vi "get active handles.vi"(8 "error in (no error)":errorcluster, 11 "Hamamatsu Camera in":refnum<class "Hamamatsu Camera.lvclass">) -> (0 "error out":errorcluster, 1 "Active Cameras":T1[](array[typedef]), 2 "Handles":u32[](array[numeric]), 3 "Hamamatsu Camera out":refnum<class "Hamamatsu Camera.lvclass">, 5 "Camera Names":string[](array[string]))   [LabVIEW 2018, in "Hamamatsu Camera.lvlib" / "Hamamatsu Camera.lvclass"]
uses:
  Hamamatsu Camera.lvclass
  Resources/Type Defs/Physical Camera Assignment.ctl
  Resources/Type Defs/Camera Type.ctl
  Hamamatsu Camera.lvclass/Hamamatsu Camera.ctl
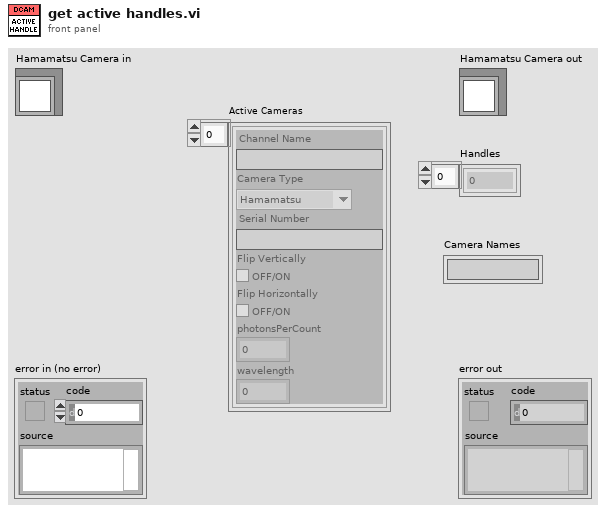
[diagram p1: front panel]
types:
  T1 = typedef "Physical Camera Assignment.ctl" = cluster{"Channel Name":string, "Camera Type":T2, "Serial Number":string, "Flip Vertically":bool, "Flip Horizontally":bool, "photonsPerCount":dbl, "wavelength":i16}
  T2 = typedef "Camera Type.ctl" = enum16{"Hamamatsu"}
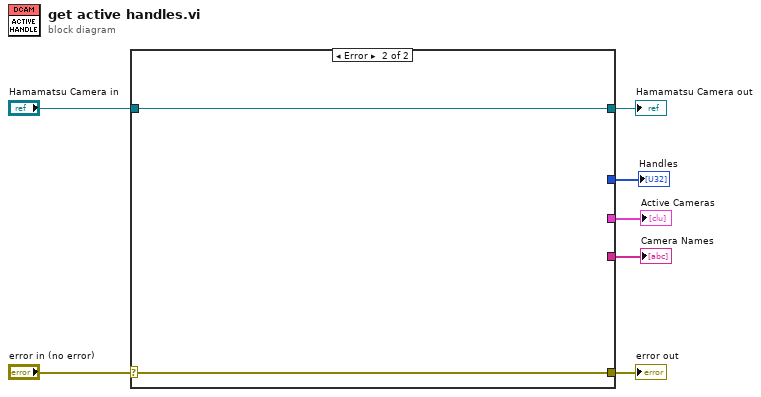
[diagram p0: block diagram]
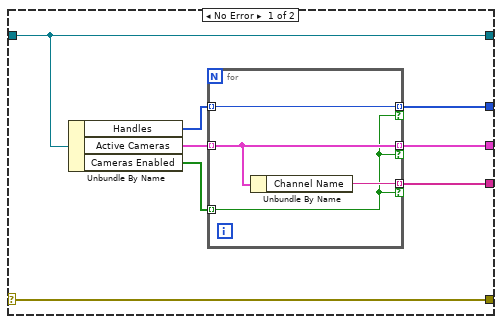
[diagram p2: hidden frame]
diagram:
  n1 = case shown="Error" "error in (no error)" {
    selector: "error in (no error)" -> [w15 w21]
    tunnel: [w15 w21] -> w6
    tunnel: [w14 w20] -> w4
    tunnel: "Hamamatsu Camera in" -> [w14 w20]
    tunnel: [w10 _] -> w3
    tunnel: [w9 _] -> w2
    tunnel: [w8 _] -> w1
    frame No Error {
      n2 = Unbundle By Name(w14) -> ("Handles"=w13:u32[], "Active Cameras"=w12:T1[], "Cameras Enabled"=w11:bool[])
      n3 = for {
        tunnel: w13 -> [w19] mode=indexing
        tunnel: w12 -> [w18] mode=indexing
        tunnel: w11 -> [w16] mode=indexing
        tunnel: [w18] -> w9 mode=indexing if=w16
        tunnel: [w19] -> w10 mode=indexing if=w16
        tunnel: [w17] -> w8 mode=indexing if=w16
        n4 = Unbundle By Name(w18) -> ("Channel Name"=w17:string)
      }
    }
    frame Error {
    }
  }
  "error out" <- w6
  "Hamamatsu Camera out" <- w4
  "Handles" <- w3
  "Active Cameras" <- w2
  "Camera Names" <- w1
